vi "sound.vi"(8 "error in (no error)":errorcluster caption="错误输入（无错误）", 10 "sound":T1(ring)) -> (0 "error out":errorcluster caption="错误输出")   [LabVIEW 2016]
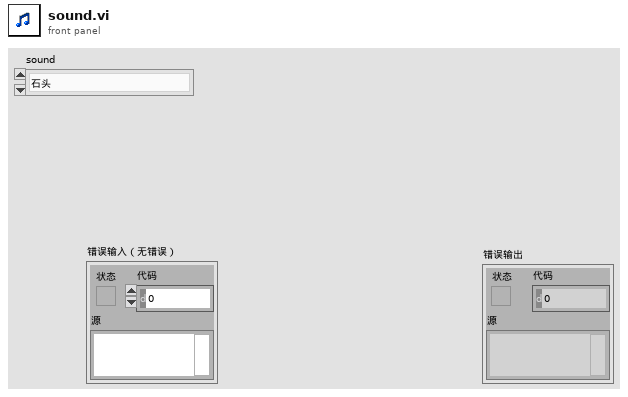
[diagram p1: front panel]
types:
  T1 = enum16{"石头", "剪刀", "布", "你赢了", "你输了", "再来一局", "NAN"}
  T2 = typedef "Sound Output Task ID.ctl" = u32
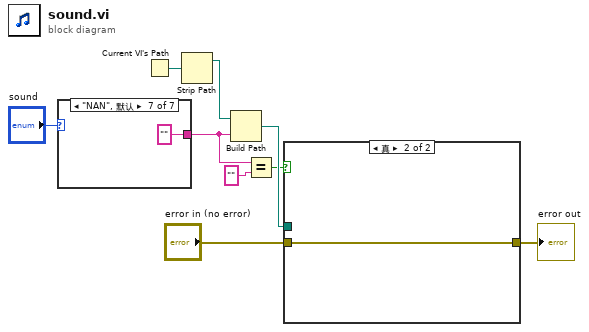
[diagram p0: block diagram]
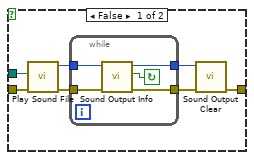
[diagram p2: hidden frame]
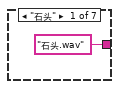
[diagram p3: hidden frame]
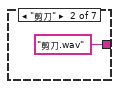
[diagram p4: hidden frame]
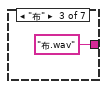
[diagram p5: hidden frame]
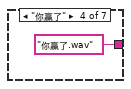
[diagram p6: hidden frame]
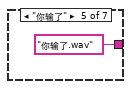
[diagram p7: hidden frame]
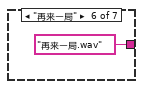
[diagram p8: hidden frame]
diagram:
  n1 = case shown="\"NAN\", 默认" "sound" {
    tunnel: ["石头.wav" ("名称或相对路径") "剪刀.wav" ("名称或相对路径") "布.wav" ("名称或相对路径") "你赢了.wav" ("名称或相对路径") "你输了.wav" ("名称或相对路径") "再来一局.wav" ("名称或相对路径") "" ("名称或相对路径")] -> w1
    frame "石头" {
    }
    frame "剪刀" {
    }
    frame "布" {
    }
    frame "你赢了" {
    }
    frame "你输了" {
    }
    frame "再来一局" {
    }
    frame "NAN", Default {
    }
  }
  n2 = Current VI's Path() -> (path=w9:path)
  n3 = Strip Path(path=w9) -> (stripped path=w3:path)  [unwired: 1 out]
  n4 = Build Path(base path=w3, name or relative path=w1) -> (appended path=w8:path)
  n5 = Equal?(x=w1, y="" ("名称或相对路径")) -> (x = y?=w4:bool)
  n6 = case shown="真" w4 {
    tunnel: "error in (no error)" -> [w19 w29]
    tunnel: [w18 w29] -> w6
    tunnel: w8 -> [w17 _]
    frame False {
      n7 = call <vilib>:"Play Sound File.vi"("error in (no error)"=w19, "path"=w17) -> ("error out"=w22:errorcluster, "task ID"=w23:T2)  [unwired: 8 in]
      n8 = while {
        tunnel: w23 -> [w27]
        tunnel: w22 -> [w26]
        tunnel: [w25] -> w21
        tunnel: [w24] -> w20
        stop <- w28 continue-if-true
        n9 = call <vilib>:"Sound Output Info.vi"("error in (no error)"=w26, "task ID"=w27) -> ("error out"=w24:errorcluster, "is playing?"=w28:bool, "task ID out"=w25:T2)  [unwired: 6 in, 1 out]
      }
      n10 = call <vilib>:"Sound Output Clear.vi"("error in (no error)"=w20, "task ID"=w21) -> ("error out"=w18:errorcluster)  [unwired: 9 in]
    }
    frame True {
    }
  }
  "error out" <- w6
